vi "DPT GET NI Data.vi"(7 "NI Card Settings":T1, 8 "Error In":errorcluster, 11 "Tasks In":refnum<k21>[](array[refnum])) -> (0 "Error Out":errorcluster, 3 "cDAQ Data":string[][](array[string]))   [LabVIEW 2020]
uses:
  Washer DOE/Type Definitions/DOE Dryer NI Card Settings.ctl
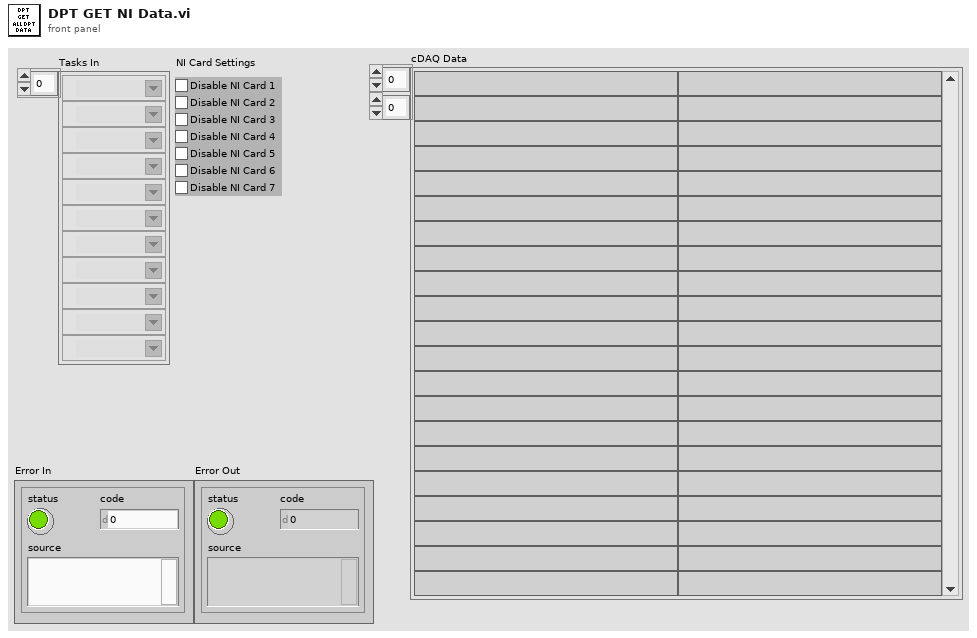
[diagram p1: front panel]
types:
  T1 = typedef "DOE Dryer NI Card Settings.ctl" = cluster{"Disable NI Card 1":bool, "Disable NI Card 2":bool, "Disable NI Card 3":bool, "Disable NI Card 4":bool, "Disable NI Card 5":bool, "Disable NI Card 6":bool, "Disable NI Card 7":bool}
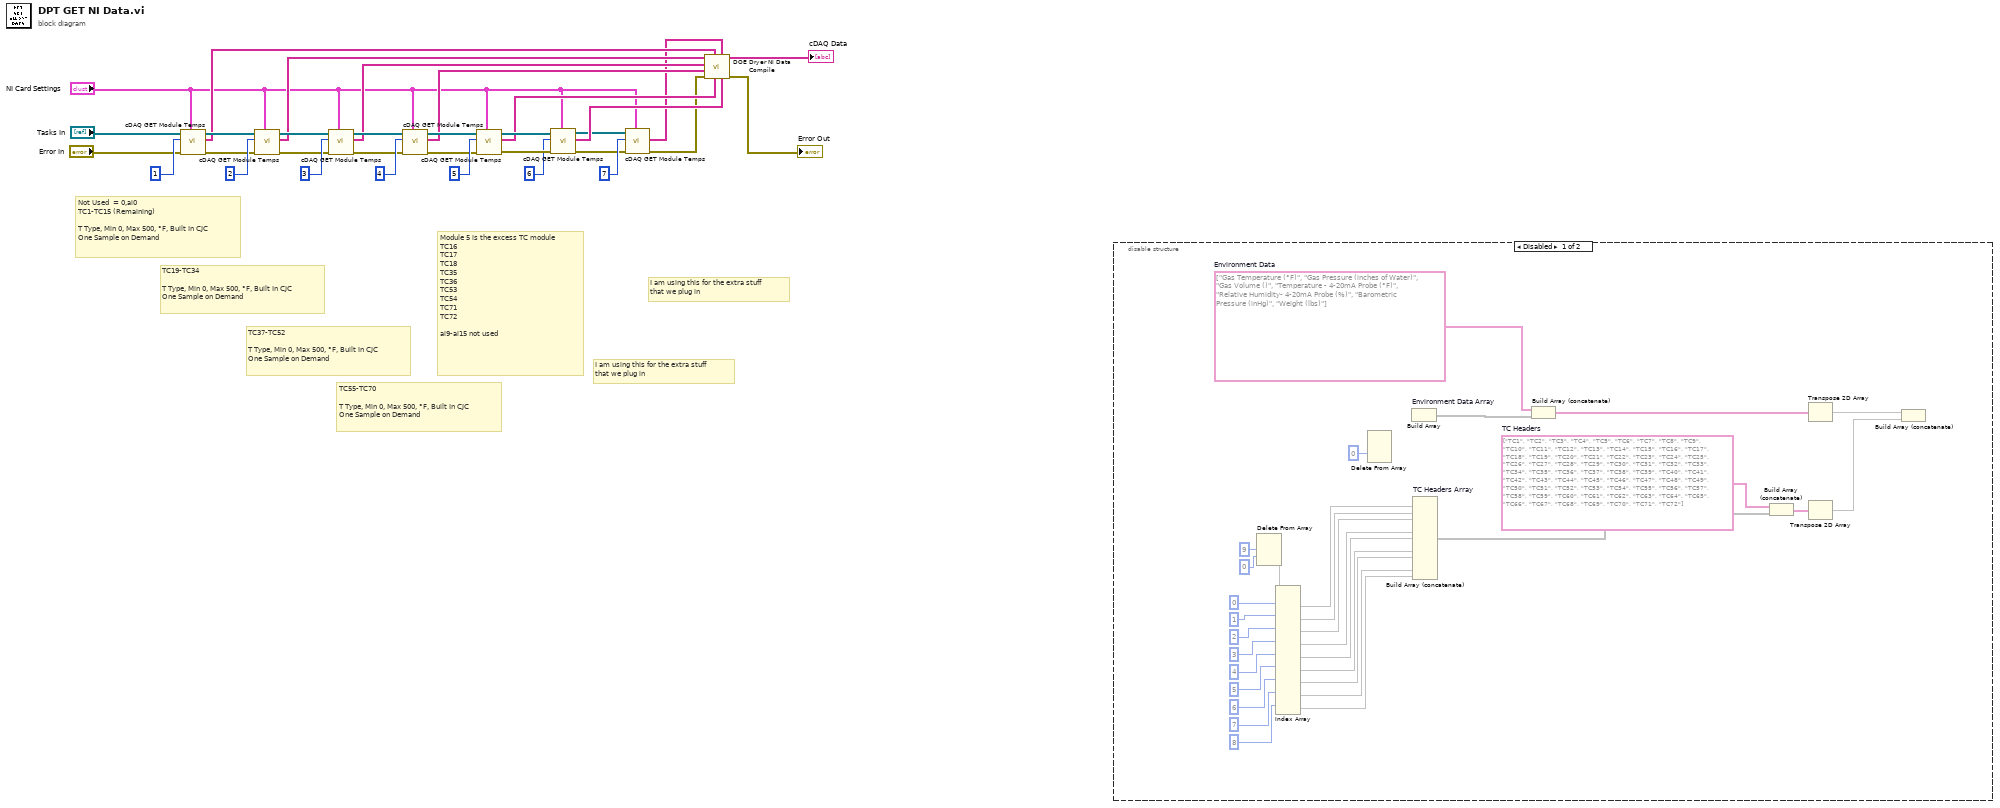
[diagram p0: block diagram]
diagram:
  # "I am using this for the extra stuff \nthat we plug in"
  # "I am using this for the extra stuff \nthat we plug in"
  # "TC55-TC70\n\nT Type, Min 0, Max 500, °F, Built In CJC\nOne Sample on Demand"
  # "TC37-TC52\n\nT Type, Min 0, Max 500, °F, Built In CJC\nOne Sample on Demand"
  # "TC19-TC34\n\nT Type, Min 0, Max 500, °F, Built In CJC\nOne Sample on Demand"
  # "Not Used  = 0,ai0\nTC1-TC15 (Remaining)\n\nT Type, Min 0, Max 500, °F, Built In CJC\nOne Sample on Demand"
  # "Module 5 is the excess TC module\nTC16\nTC17\nTC18\nTC35\nTC36\nTC53\nTC54\nTC71\nTC72\n\nai9-ai15 not used"
  n1 = call "cDAQ GET Module Temps.vi"("NI Card Settings"="NI Card Settings", "error in (no error)"="Error In", "Module Number"=1 ("index"), "Tasks (In)"="Tasks In") -> ("error out"=w27:errorcluster, "NI Module Data"=w14:string[][], "Tasks (Out)"=w21:refnum<k21>[])  [unwired: 4 in, 1 out]
  n2 = call "cDAQ GET Module Temps.vi"("NI Card Settings"="NI Card Settings", "error in (no error)"=w27, "Module Number"=2 ("Task Index"), "Tasks (In)"=w21) -> ("error out"=w26:errorcluster, "NI Module Data"=w13:string[][], "Tasks (Out)"=w19:refnum<k21>[])  [unwired: 4 in, 1 out]
  n3 = call "cDAQ GET Module Temps.vi"("NI Card Settings"="NI Card Settings", "error in (no error)"=w26, "Module Number"=3 ("Task Index"), "Tasks (In)"=w19) -> ("error out"=w25:errorcluster, "NI Module Data"=w12:string[][], "Tasks (Out)"=w18:refnum<k21>[])  [unwired: 4 in, 1 out]
  n4 = call "cDAQ GET Module Temps.vi"("NI Card Settings"="NI Card Settings", "error in (no error)"=w25, "Module Number"=4 ("Task Index"), "Tasks (In)"=w18) -> ("error out"=w24:errorcluster, "NI Module Data"=w11:string[][], "Tasks (Out)"=w17:refnum<k21>[])  [unwired: 4 in, 1 out]
  n5 = call "cDAQ GET Module Temps.vi"("NI Card Settings"="NI Card Settings", "error in (no error)"=w24, "Module Number"=5 ("Task Index"), "Tasks (In)"=w17) -> ("error out"=w23:errorcluster, "NI Module Data"=w10:string[][], "Tasks (Out)"=w16:refnum<k21>[])  [unwired: 4 in, 1 out]
  n6 = call "cDAQ GET Module Temps.vi"("NI Card Settings"="NI Card Settings", "error in (no error)"=w23, "Module Number"=6, "Tasks (In)"=w16) -> ("error out"=w5:errorcluster, "NI Module Data"=w9:string[][], "Tasks (Out)"=w3:refnum<k21>[])  [unwired: 4 in, 1 out]
  n7 = call "cDAQ GET Module Temps.vi"("NI Card Settings"="NI Card Settings", "error in (no error)"=w5, "Module Number"=7, "Tasks (In)"=w3) -> ("error out"=w4:errorcluster, "NI Module Data"=w1:string[][])  [unwired: 4 in, 2 out]
  n8 = call "DOE Dryer NI Data Compile.vi"("Module Data 6"=w9, "Module Data 7"=w1, "Module Data 5"=w10, "Module Data 1"=w14, "Error In"=w4, "Module Data 4"=w11, "Module Data 3"=w12, "Module Data 2"=w13) -> ("Error Out"=→"Error Out":errorcluster, "Data Output"=→"cDAQ Data":string[][])  [unwired: 2 in]
  n9 = disable-structure shown="Disabled" {
    frame Disabled {
      w40 = string[] ["Gas Temperature (°F)", "Gas Pressure (inches of Water)", "Gas Volume ()", "Temperature - 4-20mA Probe (°F)", "Relative Humidity- 4-20mA Probe (%)", "Barometric Pressure (inHg)", "Weight (lbs)"]  # Environment Data
      w38 = string[] ["TC1", "TC2", "TC3", "TC4", "TC5", "TC6", "TC7", "TC8", "TC9", "TC10", "TC11", "TC12", "TC13", "TC14", "TC15", "TC16", "TC17", "TC18", "TC19", "TC20", "TC21", "TC22", "TC23", "TC24", "TC25", "TC26", "TC27", "TC28", "TC29", "TC30", "TC31", "TC32", "TC33", "TC34", "TC35", "TC36", "TC37", "TC38", "TC39", "TC40", "TC41", "TC42", "TC43", "TC44", "TC45", "TC46", "TC47", "TC48", "TC49", "TC50", "TC51", "TC52", "TC53", "TC54", "TC55", "TC56", "TC57", "TC58", "TC59", "TC60", "TC61", "TC62", "TC63", "TC64", "TC65", "TC66", "TC67", "TC68", "TC69", "TC70", "TC71", "TC72"]  # TC Headers
      n10 = Delete From Array(length=9, index (row)=0 ("index")) -> (deleted portion=w41)  [unwired: 2 in, 1 out]
      n11 = Index Array(array=w41, index (row) #1=0 ("index"), index (row) #2=1 ("index"), index (row) #3=2 ("index"), index (row) #4=3 ("index"), index (row) #5=4 ("index"), index (row) #6=5 ("index"), index (row) #7=6 ("index"), index (row) #8=7 ("index"), index (row) #9=8 ("index")) -> (element #1=w58, element #2=w57, element #3=w56, element #4=w53, element #5=w52, element #6=w49, element #7=w48, element #8=w45, element #9=w44)  [unwired: 9 in]
      n12 = Delete From Array(index (row)=0 ("index")) -> ()  [unwired: 3 in, 2 out]
      n13 = Build Array "Environment Data Array"() -> (w39:void[])  [unwired: 2 in]
      n14 = Build Array (concatenate) "TC Headers Array"(w58, w57, w56, w53, w52, w49, w48, w45, w44) -> (w37:void[])  [unwired: 4 in]
      n15 = Build Array (concatenate)(w40, w39) -> (w36:string[][])
      n16 = Build Array (concatenate)(w38, w37) -> (w35:string[][])
      n17 = Transpose 2D Array(2D array=w36) -> (transposed array=w34:string[][])
      n18 = Transpose 2D Array(2D array=w35) -> (transposed array=w33:string[][])
      n19 = Build Array (concatenate)(w34, w33) -> ()  [unwired: 1 out]
    }
    frame Enabled {
    }
  }
